vi "configREFfilter.vi"(7 "address":string, 8 "error in (no error)":errorcluster, 11 "REF filter":T1={"TC (s)"=0.3, "order"=2} {"TC (s)" format="%#_6p"}) -> (0 "error out":errorcluster, 3 "REF filter":T1={"TC (s)"=0.3, "order"=2} {"TC (s)" format="%#_6p"})   [LabVIEW 2016]
doc: "API to configure the REF.\n\nIf address=\"\", this API reads from localhost\nIf address is remote lockin, you need to add this computer to allowed whitelist on the lockin computer you are trying to access."
uses:
  Typedefs/REF filter-cluster.ctl
  RemoteControl/Typedefs/Remote-SMO-Commands-Enum.ctl
  RemoteControl/LockinRemoteControl.lvclass
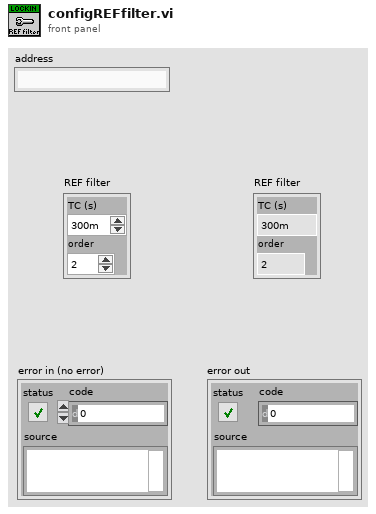
[diagram p1: front panel]
types:
  T1 = typedef "REF filter-cluster.ctl" = cluster{"TC (s)":dbl, "order":i32}
  T2 = typedef "LockinRemoteControl.lvclass/Remote-SMO-Commands-Enum.ctl" = enum16{"configAO", "configREF", "configREFfilter", "configIVmode", "configRemote", "configReset", "assertTrigger", "getAO", "getAI", "getResults", "getTrigger", "getIVmode", "getAOconfig", "getREFconfig", "getREFfilter", "ACK", "UNK", "CLOSE"}
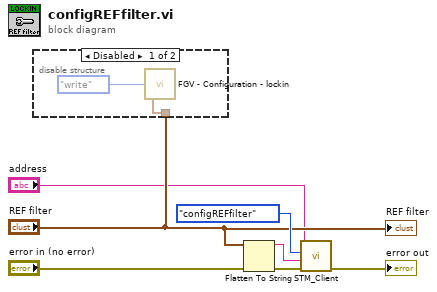
[diagram p0: block diagram]
diagram:
  n1 = disable-structure shown="Disabled" {
    disable-tunnel: "REF filter" -> [w8 _]
    frame Disabled {
      n2 = call "FGV - Configuration - lockin.vi"("Function"=enum16{"write", "read"}."write", "Channels: Lockin"=w8) -> ()  [unwired: 4 in, 2 out]
    }
    frame Enabled {
    }
  }
  n3 = Flatten To String(anything="REF filter", error in (no error)="error in (no error)") -> (data string=w6:string, error out=w7:errorcluster)  [unwired: 2 in, 1 out]
  n4 = call "STM_Client.vi"("error in (no error)"=w7, "data to send"=w6, "Command"=Remote-SMO-Commands-Enum."configREFfilter", "address"="address") -> ("error out"=→"error out":errorcluster)  [unwired: 6 in, 1 out]
  "REF filter" <- "REF filter"
